vi "AlliGator Get Python Plugin Function Parameters String.vi"(8 "error in (no error)":errorcluster, 10 "Function Parameters":T1[](array[typedef]), 11 "Function Display Name":string) -> (0 "error out":errorcluster, 2 "Function Parameters JSON String":string, 3 "Parameter Names Not Found":string[](array[string]))   [LabVIEW 2021, in "AlliGator Python Plugins.lvlib"]
doc: "Gets requested parameter names from the python function description, opens up a dialog window to allow the user to enter the required parameters, and builds a JSON string to pass those parameters (names and values) to the python function."
uses:
  AlliGator Python Plugins.lvlib
  AlliGator Python Function Parameter Definition.ctl
  Globals, Variables, Constants/AlliGator Variables List.ctl
  d4008f8b-8ee3-446b-8e9c-2fee3dc7eda3.vi
  <userlib>/_OpenG.lib/string/string.llb/To Proper Case (String)__ogtk.vi
  <vilib>/JDP Science/JSONtext/Variant to JSON Text.vi
  <vilib>/JDP Science/JSONtext/support/Format JSON Object.vi
  <vilib>/JDP Science/JSONtext/LVClass Serializer/JSONtext LVClass Serializer.lvclass
  Settings/AlliGator Settings.lvlib
  Globals, Variables, Constants/AlliGator Globals, Variables & Constants.lvlib
  <vilib>/JDP Science/JSONtext/JSONtext.lvlib
  <userlib>/_OpenG.lib/string/string.llb/openg_string.lvlib
panel:
  # "see the AlliGator License on the block diagram (Ctrl+E or Window:Show Block Diagram)"
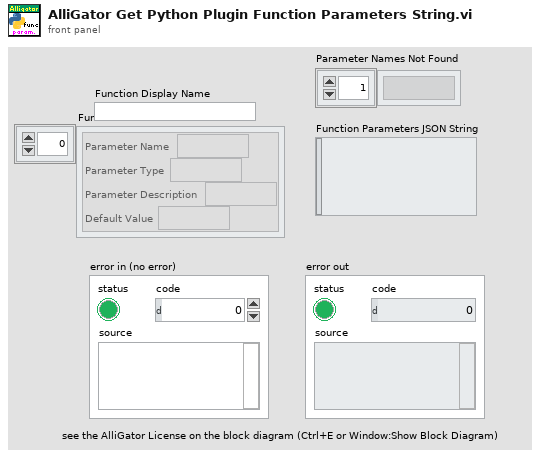
[diagram p1: front panel]
types:
  T1 = typedef "AlliGator Python Plugins.lvlib/AlliGator Python Function Parameter Definition.ctl" = cluster{"Parameter Name":string, "Parameter Type":string, "Parameter Description":string, "Default Value":string}
  T2 = typedef "AlliGator Globals, Variables & Constants.lvlib/AlliGator Variables List.ctl" = enum16{"---- GUI ----", "GUI:Initialization Status", "GUI:State Indicators Refnum", "GUI:Original AlliGator Menu Items", "GUI:Current Action Loop State", "GUI:Script in progress", "GUI:Playback", "GUI:Loop Playback", "GUI:Search ROI Used", "GUI:Search ROI", "Decay Graph Max Legend Size", "Intensity Graph Max Legend Size", "Decay Statistics Graph Max Legend Size", "Phasor Graph Max Legend Size", "Phasor Ratio Graph Max Legend Size", "Lifetime Graph Max Legend Size", "---- Files ----", "Files:Export Dataset Frames as Individual Files", "Files:Show Batch Export Help Balloons", "Files:Frames in Dataset", "Files:ptu File Frame Start Indices", "Files:Current Frame in Dataset", "Files:Current Frame Timestamp", "Files:Dataset Loaded", "Files:Dataset Metadata", "Files:Dataset Channel", "Files:Dataset Data Description", "Files:Background Dataset Metadata", "Files:Background Dataset Channel", "Files:Background Dataset Data Description", "Files:Background File Subtraction", "Files:Background File Path", "Files:Background File Pile-up Correction", "Files:Background File Pixel Well Capacity", "Files:Background File Scaling Factor", "Files:Current Dataset Load Settings", "Files:Dataset Path", "Files:ICCD-specific Information", "Files:Macrotime Gate Separation", "------ Python Plugins ------", "Python Plugins:Information", "Python Plugins:Python Session", "Python Plugins:Valid Python Session?", "---- Source Image ----", "Source Image:ROIs", "Source Image:Current ROI", "Source Image:ROI Event Refnum", "X_Source Image:Display Range", "X_Source Image:Palette Information", "X_Source Image:Type of Displayed Image", "X_Time Gate Slider", "Source Image:Palette List", "Source Image:Scale", "Source Image:ROI Overlay Color", "Source Image:Overlay to Erase", "Source Image:Is Displayed Image Accumulated", "Source Image:White Light Image Modified", "Source Image:Mask Image Modified", "---- Image Profile Window ----", "Image Profile:Window Event Refnum", "Image Profile:IntensityType", "Image Profile:Intensity Average Type", "Image Profile:Intensity-weighted SDV", "Image Profile:Box Profile Type", "Image Profile:Window Open", "Image Profile:Plotted Fit Parameter", "------ Phasor Graph -------", "Phasor Graph:Show Line", "---- Phasor Plot ---", "Phasor Plot:Parameters Changed", "Phasor Plot:FLI Dataset Modified since last Calculation", "Phasor Harmonics Data", "Selected Phasor Harmonics", "Phasor Harmonic Manager Event Refnum", "Phasor Plot:ROIs", "Phasor Plot:Current ROI", "Phasor Plot:ROI Event Refnum", "Phasor Plot:Image Reference Points", "Phasor Plot:Computed", "Phasor Plot:Palette Information", "Phasor Plot:Palette List", "Phasor Plot:Phasor Ratio Palette Information", "Phasor Plot:Phasor Ratio Palette List", "Phasor Plot:Image Scale", "Phasor Plot:Image Overlay to Erase", "Phasor Plot:Image Elements to Update", "Phasor Plot:Current Calculation Parameters", "Phasor Plot:Current Calibration Options", "Phasor Plot:Reset Cumulated Phasor Plot", "Phasor Plot:Reference 1", "Phasor Plot:Lifetime Reference 1", "Phasor Plot:Reference 1 Frequency", "Phasor Plot:Reference 2", "Phasor Plot:Lifetime Reference 2", "Phasor Plot:Reference 2 Frequency", "---- Decay Analysis ----", "Number of Selected Decays to Fit", "LS Fit Results", "LAR Fit Results", "BS Fit Results", "Last Decay Max - Min", "Best Fit Parameters", "Best Fit Parameter Names", "Actual Size X", "Actual Size Y", "Binning X", "Binning Y", "Actual # Gates", "Dataset Number", "Gates to...", "Gates Skipped", "Gates to keep", "Gate Step", "Gate Separation", "Reversed Gates", "Pile-up Correction", "Pixel Well Capacity", "Background Subtracted", "Background Subtraction Method", "Background Definition Range", "Background File (deprecated)", "Number of Dataset Accumulated", "Array of Accumulated Dataset Paths", "Do Averaged Datasets", "Destination File Path", "Process Plot Target", "Use 1/D as Phasor Frequency", "---- Decay Fit Parameter Map -----", "Decay Fit Parameter Map:Palette Information", "Decay Fit Parameter Map:Palette List", "Decay Fit Parameter Map:X Resolution", "Decay Fit Parameter Map:Y Resolution", "Decay Fit Parameter Map:Use Decay Fit Result Constraints", "Decay Fit Parameter Map:Decay Fit Result Constraints", "Decay Fit Parameter Map:Decay Fit Result Constraints Applied", "---- Parameter Map ----", "Parameter Map:Palette Information", "Parameter Map:Palette List", "------- Local Decay Window ---------", "Local Decay Graph Window:Event Refnum", "Local Decay Graph Window:Use normalized IRF for convolution", "----- Miscellaneous ----", "Misc:Skippable Dialog Windows Status"}
  T3 = typedef "AlliGator Settings.lvlib/AlliGator Settings List.ctl" = enum16{"GUI:Visible Settings Tab", "GUI:Last Run Version", "Source Image:Use Image Histogram for Contrast", "Source Image:Low Count Pixels Rejection Options", "Source Image:High Count Pixels Rejection Options", "Source Image:Use Image Brightness", "Source Image:Blend Overlay with Image Background", "Source Image:Use Fixed ROI Diameter", "Source Image:ROI Diameter", "Source Image:ROI Center Color", "Source Image:Peak Threshold", "Source Image:Intensity Threshold", "Source Image:Image Binning Options", "Source Image:Image Smoothing Options", "Source Image:Image Histogram Active", "Source Image:Invert Binary Mask", "Source Image:Hot Pixel Removal", "Source Image:Overlay Analyzed ROI Center", "Source Image:Auto-Adjust Contrast", "Source Image:Histogram Lower Percentile", "Source Image:Histogram Upper Percentile", "Source Image:Save Source Image", "Source Image:Scale Bar Options", "Source Image:Image Resolution (Pixel Size)", "Source Image:Flatfield Correction", "Source Image:Show Dead Left Columns Correction", "Source Image:Dead Left Columns Correction", "Source Image:Image Pre-Processing Operations Order", "Source Image:Overlay ROI Median", "Source Image:Median Overlay Color", "Data Information:Gate Width", "Data Information:Nanotime Gate Separation", "Data Information:Macrotime Gate Separation", "Data Information:Gate Step", "Data Information:# Gates", "Data Information:Gate Image Exposure", "Data Information:Gate Image Integration", "Data Information:Gates to Skip", "Data Information:Gates to Keep", "Data Information:Define Gates to", "Data Information:Channel Name", "Data Information:Available Channel Names", "Data Information:Channel Arithmetic", "Data Information:Background File Subtraction", "Data Information:Background File", "Data Information:Background Scaling Factor", "Data Information:Background Pile-up Correction", "Data Information:Background Pixel Well Capacity", "Data Information:Laser Period", "Data Information:SYNC Period", "Data Information:Pile-up Correction", "Data Information:Pixel Well Capacity", "Data Information:Dataset Scaling Factor", "Fluorescence Decay_Decay Pre-Processing:Reverse Gates", "Fluorescence Decay_Decay Pre-Processing:Verbose Decay Pre-Processing", "Fluorescence Decay_Decay Pre-Processing:Use Decay Pre-Processing", "Fluorescence Decay_Decay Pre-Processing:Background Subtraction", "Fluorescence Decay_Decay Pre-Processing:Background Definition Range", "Fluorescence Decay_Decay Pre-Processing:Baseline Subtraction Method", "Fluorescence Decay_Decay Pre-Processing:Decay Pre-Processing Operations Order", "Fluorescence Decay_Decay Pre-Processing:Smoothing Parameter", "Fluorescence Decay_Decay Pre-Processing:Shift Decay", "Fluorescence Decay_Decay Pre-Processing:Decay Shift Parameters", "Fluorescence Decay_Decay Pre-Processing:Fold Decay", "Fluorescence Decay_Decay Pre-Processing:# Folds", "Fluorescence Decay_Decay Pre-Processing:1-Normalize Decay", "Fluorescence Decay_Decay Pre-Processing:[0-1]-Normalize Decay", "Fluorescence Decay_Decay Pre-Processing:Smoothen Decay", "Fluorescence Decay_Decay Pre-Processing:Extrapolate Decay", "Fluorescence Decay_Decay Pre-Processing:Use Periodicity", "Fluorescence Decay_Decay Pre-Processing:Use Cursors", "Fluorescence Decay_Decay Pre-Processing:Tail Fraction", "Fluorescence Decay_Decay Pre-Processing:Head Fraction", "Fluorescence Decay_Decay Pre-Processing:Additional Points", "Fluorescence Decay_Decay Pre-Processing:Straighten Decay", "Fluorescence Decay_Decay Pre-Processing:Constant Background", "Fluorescence Decay_Decay Pre-Processing:Pixel-Normalize Decay", "Fluorescence Decay_Advanced Analysis:Extract IRF instead of Decay", "Fluorescence Decay_Advanced Analysis:IRF Extraction Options", "Fluorescence Decay_Advanced Analysis:IRF Optimization Options", "Fluorescence Decay_Advanced Analysis:Square Pulse Options", "Fluorescence Decay_Advanced Analysis:IRF Order", "Fluorescence Decay_Advanced Analysis:IRF Time Constants", "Fluorescence Decay_Advanced Analysis:Wavelet Analysis Options", "Fluorescence Decay_Advanced Analysis:Average Lifetime Options", "Fluorescence Decay_Fit Options:Fit Options", "Fluorescence Decay_Fit Options:Use Legacy Fitting Approach", "Fluorescence Decay_Fit Options:Use Data Information Laser Period", "Fluorescence Decay_Fit Parameters:Displayed Fit Parameters", "Fluorescence Decay_Fit Parameters:Fit Parameter Constraints", "Fluorescence Decay_Fit Parameters:Export Tabulated Results", "Fluorescence Decay_Fit Parameters:MLE Baseline Offset Type", "Fluorescence Decay_Fit Parameters:MLE Baseline Offset", "Fluorescence Decay_Fit Parameters:Guess Parameter Names", "Fluorescence Decay_Fit Parameters:Guess Parameter Values", "Fluorescence Decay_Fit Parameters:Guess Parameters Options", "Fluorescence Decay_Fit Parameters:Optimal Offset Selection Criterion", "Fluorescence Decay_Styles:Show Last Decay Only", "Fluorescence Decay_Styles:Decay Graph Color Array", "Fluorescence Decay:Decay Graph Active", "Fluorescence Decay Statistics:Min Peak Value", "Fluorescence Decay Statistics:Reject Low Decay Peak Pixels", "Fluorescence Decay Statistics:Reject High Decay Peak Pixels", "Fluorescence Decay Statistics:Max Peak Value", "Time Traces:Use File Timestamp", "Time Traces:Time Step", "Time Traces:Use Intensity Correction File", "Time Traces:Intensity Correction File", "Phasor Plot:Phasor Plot Smoothing Options", "Phasor Plot:Phasor Plot Size", "Phasor Plot:Phasor Plot Graphics Options", "Phasor Plot:Cumulative Phasor Plot", "Phasor Plot:Use Phasor Brightness", "Phasor Plot:Blend Overlay with Phasor Background", "Phasor Plot:Save Phasor Plot", "Phasor Plot:Show References", "Phasor Plot:Phasor Ratio Decay Range", "Phasor Plot:Exponential Fading", "Phasor Plot:Phasor Ratio Reference Colors", "Phasor Plot:Reference Radius", "Phasor Plot:Show Color Map Vertices", "Phasor Plot:Phasor Plot Active", "Phasor Plot:Phasor Ratio Color Map Type", "Phasor Plot:Phasor Ratio Color Map", "Phasor Plot:Phasor Ratio Display Range", "Phasor Plot:Selected Image ROI(s)", "Phasor Plot:All Image ROIs", "Phasor Plot:Selected Phasor Plot ROI(s)", "Phasor Plot:All Phasor Plot ROIs", "Phasor Plot:Phasor Ratio Color-Coded Quantity", "Phasor Plot:Store Phasor Harmonics", "Phasor Plot:Draw Reference Segment", "Phasor Plot:User-Defined Quantity", "Phasor Plot:Color Scale High Color", "Phasor Plot:Color Scale Low Color", "Phasor Plot:Intensity-weighted Phasor Plot", "Phasor Graph:Phasor Frequency", "Phasor Graph:Phasor Ratio Type", "Phasor Graph:Pixel-level Phasor Computation", "Phasor Graph:Save Phasor Graph", "Phasor Graph:Phasor Graph Active", "Phasor Graph:Phasor SDV Options", "Phasor Graph:Intensity-weighted Phasor Graph", "Phasor Graph:Define Shortest Lifetime as", "Phasor Calibration:Use Backup Calibration if needed", "Phasor Calibration:Backup Calibration Type", "Phasor Calibration:Calibration Type", "Phasor Calibration:Calibration Lifetime", "Phasor Calibration:Calibration Map Algorithm", "Single-Exponential Phasor Locus (SEPL):Gate Parameters", "Single-Exponential Phasor Locus (SEPL):User-defined Gate", "Single-Exponential Phasor Locus (SEPL):User-defined IRF", "Single-Exponential Phasor Locus (SEPL):Phasor Parameters", "Single-Exponential Phasor Locus (SEPL):Decay & IRF Parameters", "Single-Exponential Phasor Locus (SEPL):Display Parameters", "Lifetime Analysis:Decay Analysis Parameters", "Lifetime Analysis:Lifetime Map Active", "Plugins:Python Settings", "Miscellaneous:Verbose Mode", "Miscellaneous:Beep after Script", "Miscellaneous:Saved Image File Format", "Miscellaneous:Exported Gate Image Settings", "Miscellaneous:Include Loading in Timing", "Miscellaneous:Verbose Settings Mode", "Miscellaneous:Histogram Options", "Miscellaneous:Beep on Error", "Miscellaneous:# Logical Processors Used", "Miscellaneous:ROI Description Max Characters", "Miscellaneous:Verbose Error Mode", "Miscellaneous:Transparent Mask Color"}
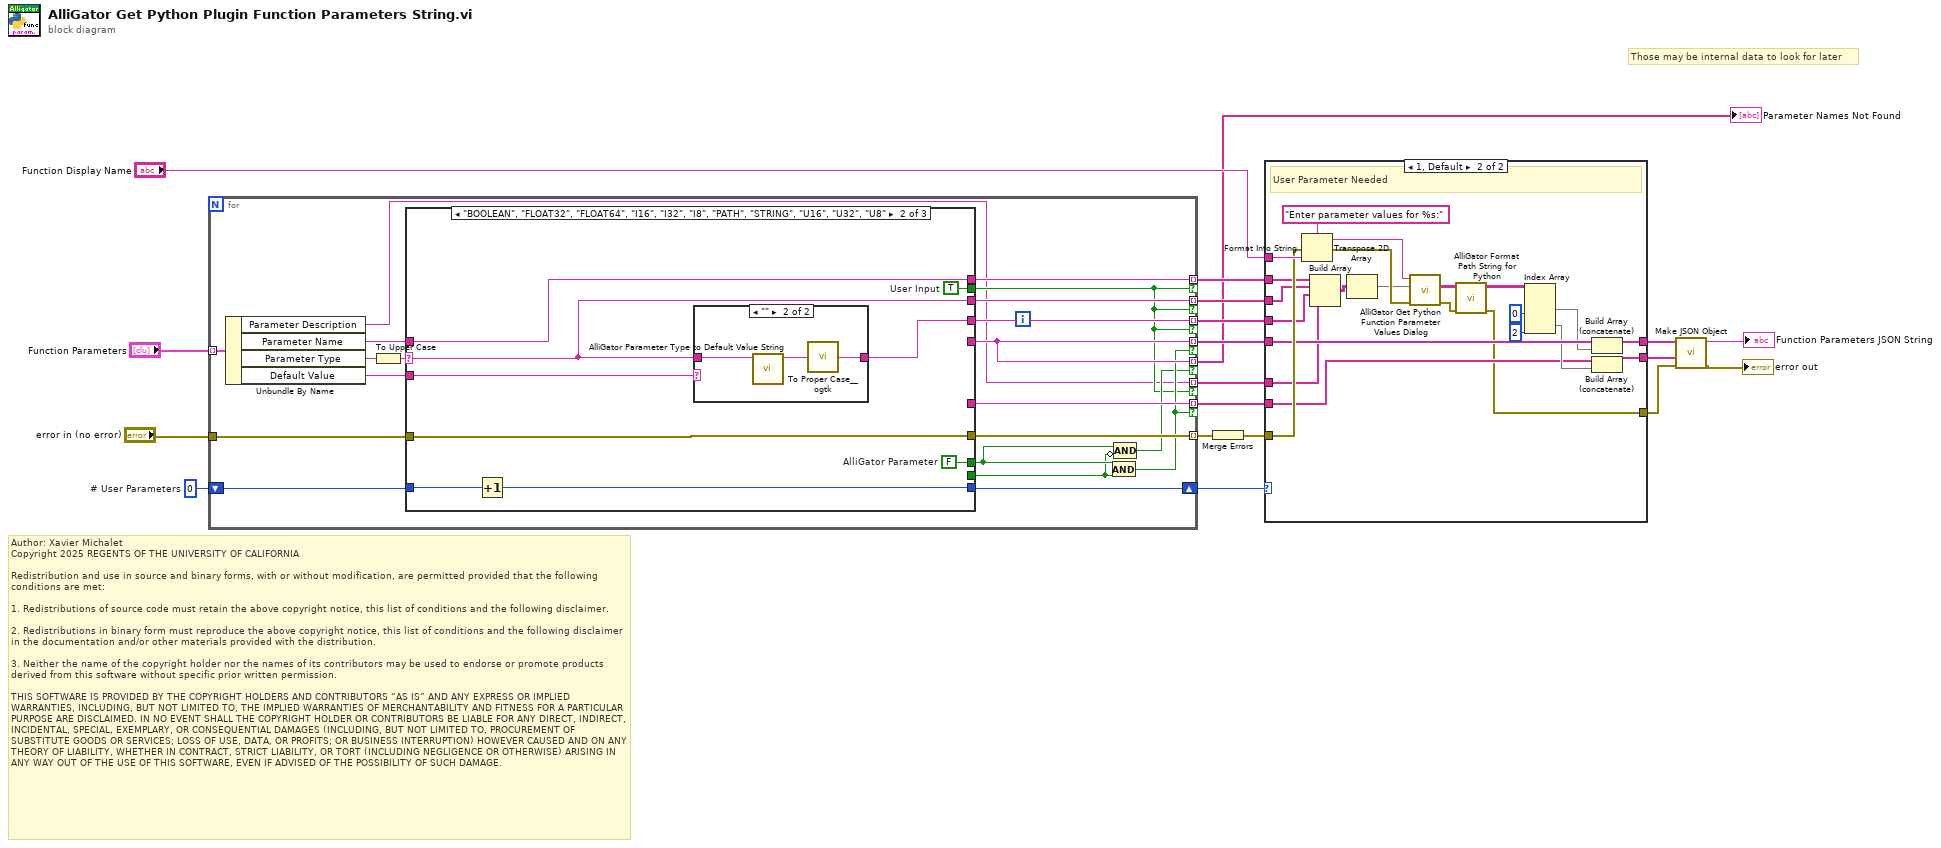
[diagram p0: block diagram]
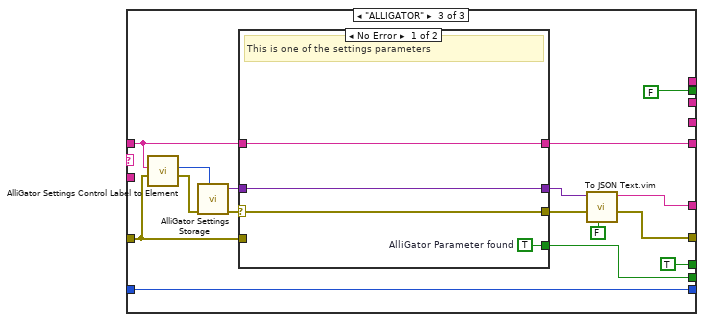
[diagram p5: hidden frame]
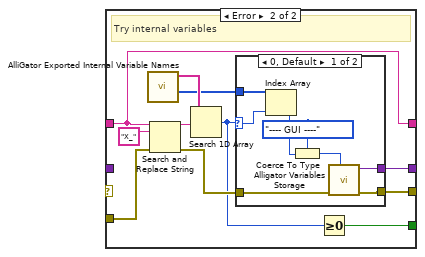
[diagram p6: hidden frame]
diagram:
  w14 = 0  # # User Parameters
  # "Author: Xavier Michalet\nCopyright 2025 REGENTS OF THE UNIVERSITY OF CALIFORNIA\n\nRedistribution and use in source and binary forms, with or without modification, are permitted provided that the following conditions are met:\n\n1. Redistributions of source code must retain the above copyright notice, this list of conditions and the following disclaimer.\n\n2. Redistributions in binary form must reproduce the above copyright notice, this list of conditions and the following disclaimer in the documentation and/or other materials provided with the distribution.\n\n3. Neither the name of the copyright holder nor the names of its contributors may be used to endorse or promote products derived from this software without specific prior written permission.\n\nTHIS SOFTWARE IS PROVIDED BY THE COPYRIGHT HOLDERS AND CONTRIBUTORS “AS IS” AND ANY EXPRESS OR IMPLIED WARRANTIES, INCLUDING, BUT NOT LIMITED TO, THE IMPLIED WARRANTIES OF MERCHANTABILITY AND FITNESS FOR A PARTICULAR PURPOSE ARE DISCLAIMED. IN NO EVENT SHALL THE COPYRIGHT HOLDER OR CONTRIBUTORS BE LIABLE FOR ANY DIRECT, INDIRECT, INCIDENTAL, SPECIAL, EXEMPLARY, OR CONSEQUENTIAL DAMAGES (INCLUDING, BUT NOT LIMITED TO, PROCUREMENT OF SUBSTITUTE GOODS OR SERVICES; LOSS OF USE, DATA, OR PROFITS; OR BUSINESS INTERRUPTION) HOWEVER CAUSED AND ON ANY THEORY OF LIABILITY, WHETHER IN CONTRACT, STRICT LIABILITY, OR TORT (INCLUDING NEGLIGENCE OR OTHERWISE) ARISING IN ANY WAY OUT OF THE USE OF THIS SOFTWARE, EVEN IF ADVISED OF THE POSSIBILITY OF SUCH DAMAGE."
  # "Those may be internal data to look for later"
  n1 = for {
    tunnel: "Function Parameters" -> [w39] mode=indexing
    tunnel: [w36] -> w18 mode=indexing
    tunnel: "error in (no error)" -> [w35]
    shift-right: [w33] -> w13
    shift-left: w14 -> [w34]
    tunnel: [w32] -> w12 mode=indexing if=w26
    tunnel: [w28] -> w11 mode=indexing if=w26
    tunnel: [w31] -> w10 mode=indexing if=w22
    tunnel: [w30] -> w9 mode=indexing if=w22
    tunnel: [w29] -> w8 mode=indexing if=w22
    tunnel: [w28] -> w2 mode=indexing if=w23
    tunnel: [w21] -> w1 mode=indexing if=w22
    n2 = Unbundle By Name(w39) -> ("Parameter Description"=w21:string, "Parameter Name"=w38:string, "Parameter Type"=w37:string, "Default Value"=w20:string)
    n3 = To Upper Case(1:w37) -> (0:w27:string)
    n4 = case shown="\"BOOLEAN\", \"FLOAT32\", \"FLOAT64\", \"I16\", \"I32\", \"I8\", \"PATH\", \"STRING\", \"U16\", \"U32\", \"U8\"" w27 {
      selector: w27 -> [_ w45 _]
      tunnel: w38 -> [_ w48 w60]
      tunnel: [w41 w47 w55] -> w36
      tunnel: w35 -> [w41 w47 w62]
      tunnel: w34 -> [w40 w50 w68]
      tunnel: [w40 w49 w68] -> w33
      tunnel: [_ _ w61] -> w32
      tunnel: [_ _ w59] -> w28
      tunnel: [_ w44 TRUE ("AlliGator Parameter")] -> w25
      tunnel: [_ w48 _] -> w31
      tunnel: [_ w45 _] -> w30
      tunnel: [_ w46 FALSE ("Pretty Print?")] -> w22
      tunnel: [_ w43 _] -> w29
      tunnel: [_ _ w56] -> w24
      tunnel: w20 -> [_ w42 _]
      frame "", Default {
      }
      frame "BOOLEAN", "FLOAT32", "FLOAT64", "I16", "I32", "I8", "PATH", "STRING", "U16", "U32", "U8" {
        w44 = FALSE  # AlliGator Parameter
        w46 = TRUE  # User Input
        n5 = Increment(x=w50) -> (x+1=w49:i32)
        n6 = case shown="\"\"" w42 {
          selector: w42 -> [w51 _]
          tunnel: w45 -> [_ w54]
          tunnel: [w51 w52] -> w43
          frame "0", Default {
          }
          frame "" {
            n7 = call "AlliGator Parameter Type to Default Value String.vi"("Parameter Type"=w54) -> ("Default Parameter String"=w53:string)  [unwired: 10 in]
            n8 = call-poly <userlib>:"To Proper Case__ogtk.vi"("string"=w53) -> ("proper case string"=w52:string)  [unwired: 4 in]
          }
        }
      }
      frame "ALLIGATOR" {
        n9 = call "AlliGator Settings Control Label to Element.vi"("Error In"=w62, "Control Label"=w60) -> ("Error Out"=w67:errorcluster, "AlliGator Settings List Element"=w70:T3)  [unwired: 6 in]
        n10 = call "AlliGator Settings Storage.vi"("AlliGator Settings List"=w70, "Error In"=w67) -> ("Error Out"=w66:errorcluster, "Variant Data out"=w65:variant)  [unwired: 8 in]
        n11 = case shown="No Error" w66 {
          selector: w66 -> [w74 _]
          tunnel: w65 -> [w73 _]
          tunnel: [w74 w85] -> w64
          tunnel: [w73 w84] -> w63
          tunnel: w62 -> [_ w82]
          tunnel: w60 -> [w72 w77]
          tunnel: [w72 w77] -> w59
          tunnel: [w71 w75] -> w56
          frame No Error {
            w71 = TRUE  # AlliGator Parameter found
            # "This is one of the settings parameters"
          }
          frame Error {
            # "Try internal variables"
            n12 = call "AlliGator Exported Internal Variable Names.vi"() -> ("Indices of Exported IVs"=w79:i32[], "Exported IV Name Array"=w81:string[])  [unwired: 10 in]
            n13 = Search and Replace String(input string=w77, search string="X_" ("replace string (\"\")"), error in=w82) -> (result string=w80:string, error out=w83:errorcluster)  [unwired: 5 in, 2 out]
            n14 = Search 1D Array(1D array=w81, element=w80) -> (index of element=w76:i32)  [unwired: 1 in]
            n15 = case shown="0, Default" w76 {
              selector: w76 -> [w87 _]
              tunnel: [w93 w94] -> w85
              tunnel: [w92 _] -> w84
              tunnel: w83 -> [w89 w94]
              tunnel: w79 -> [w88 _]
              frame 0, Default {
                n16 = Index Array(array=w88, index=w87) -> (element=w86:i32)
                n17 = Coerce To Type(0:w86, 1:AlliGator_Variables_List."---- GUI ----" ("Alligator Variable")) -> (2:w91:T2)
                n18 = call "Alligator Variables Storage.vi"("AlliGator Variable"=w91, "Error In"=w89) -> ("Error Out"=w93:errorcluster, "Data out"=w92:variant)  [unwired: 7 in, 1 out]
              }
              frame -1 {
                # "not found"
              }
            }
            n19 = Greater Or Equal To 0?(x=w76) -> (x >= 0?=w75:bool)
          }
        }
        n20 = call "To JSON Text.vim"("Pretty Print?"=FALSE, "error in (no error)"=w64, "Anything"=w63) -> ("error out"=w55:errorcluster, "<JSON>"=w61:string)  [unwired: 7 in]
      }
    }
    n21 = And(x=w25, y=w24) -> (x .and. y?=w26:bool)
    n22 = Compound Arithmetic op=AND(w25, invert w24) -> (w23:bool)
  }
  "Parameter Names Not Found" <- w2
  n23 = Merge Errors(w18) -> (w16:errorcluster)
  n24 = case shown="1, Default" w13 {
    tunnel: "Function Display Name" -> [_ w120]
    tunnel: [w97 w99] -> w7
    tunnel: w16 -> [w97 w116]
    tunnel: w12 -> [w96 w106]
    tunnel: w11 -> [w95 w110]
    tunnel: w10 -> [_ w115]
    tunnel: w9 -> [_ w114]
    tunnel: w8 -> [_ w113]
    tunnel: [w96 w105] -> w5
    tunnel: [w95 w108] -> w4
    tunnel: w1 -> [_ w98]
    frame 0 {
      # "No user-input needed"
    }
    frame 1, Default {
      # "User Parameter Needed"
      n25 = Format Into String(format string="Enter parameter values for %s:", error in=w116, w120) -> (resulting string=w118:string, error out=w117:errorcluster)  [unwired: 1 in]
      n26 = Build Array(w115, w114, w113, w98) -> (w112:string[][])
      n27 = Transpose 2D Array(2D array=w112) -> (transposed array=w102:string[][])
      n28 = call "AlliGator Get Python Function Parameter Values Dialog.vi"("Error In"=w117, "Parameters In"=w102, "Input Message"=w118) -> ("Error Out"=w100:errorcluster, "Parameters Out"=w111:string[][])  [unwired: 6 in, 1 out]
      n29 = call "AlliGator Format Path String for Python.vi"("Error In"=w100, "Python Plugin Dialog Output"=w111) -> ("Error Out"=w99:errorcluster, "Python Plugin Dialog Output"=w101:string[][])  [unwired: 8 in]
      n30 = Index Array(array=w101, index (col) #1=0 ("disabled index (col)"), index (col) #2=2 ("index (col)")) -> (element #1=w109:string[], element #2=w107:string[])  [unwired: 2 in]
      n31 = Build Array (concatenate)(w110, w109) -> (w108:string[])
      n32 = Build Array (concatenate)(w106, w107) -> (w105:string[])
    }
  }
  n33 = call <vilib>:"Make JSON Object.vi"("error in (no error)"=w7, "JSON Items"=w5, "Item Names"=w4) -> ("error out"=→"error out":errorcluster, "<JSON>"=→"Function Parameters JSON String":string)  [unwired: 7 in]
